vi "TimedTrigger.vi"(8 "error in (no error)":errorcluster, 10 "clTimedTrigger":T1={"TriggerName"="", "Time after next UTC Second"=0.0, "Trigger Duration"=0.1, "Edge"=enum."Rising"}, 11 "PXI_MultiTrig in":refnum<class "PXI_MultiTrig.lvclass">) -> (0 "error out":errorcluster, 3 "PXI_MultiTrig out":refnum<class "PXI_MultiTrig.lvclass">)   [LabVIEW 2018, in "SyncPlugins.lvlib" / "PXI_MultiTrig.lvclass"]
uses:
  PXI_MultiTrig.lvclass
  SyncPluginBase/Typedefs/clTimedTrigger.ctl
  PXI_MultiTrig.lvclass/PXI_MultiTrig.ctl
  Accessors/Read RefClkSession.vi
  Accessors/Write RefClkSession.vi
  Accessors/Write Triggers.vi
  Accessors/Read Triggers.vi
  <vilib>/Utility/error.llb/Error Cluster From Error Code.vi
  <vilib>/ErrorRing/Error Ring.xnode
  SyncPluginBase/SyncPluginBase.lvclass
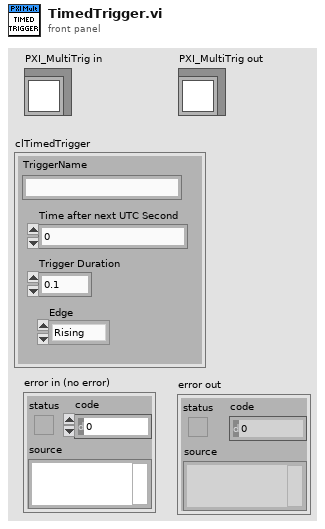
[diagram p1: front panel]
types:
  T1 = typedef "SyncPlugins.lvlib/SyncPluginBase.lvclass/clTimedTrigger.ctl" = cluster{"TriggerName":string, "Time after next UTC Second":dbl, "Trigger Duration":dbl, "Edge":enum16{"Rising", "Falling"}}
  T2 = typedef "SyncPlugins.lvlib/PXI_MultiTrig.lvclass/clTrigger.ctl" = cluster{"Name":string, "DestTerm":string, "SrcTerm":string, "SyncClk":string, "Edge":i32, "Invert?":i32, "Initiated":bool, "Type":string, "TrigTime":bool}
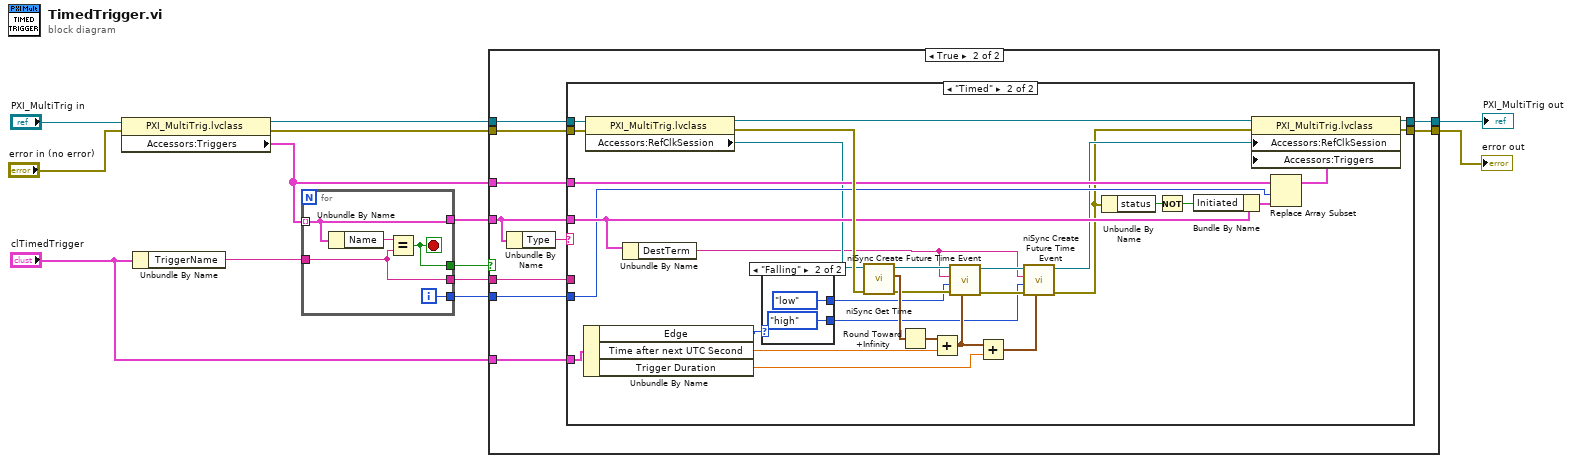
[diagram p0: block diagram]
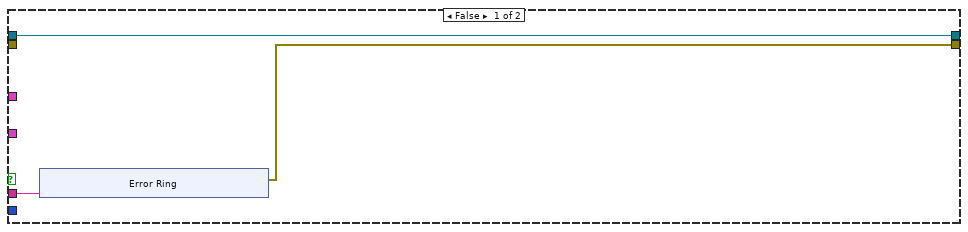
[diagram p2: hidden frame]
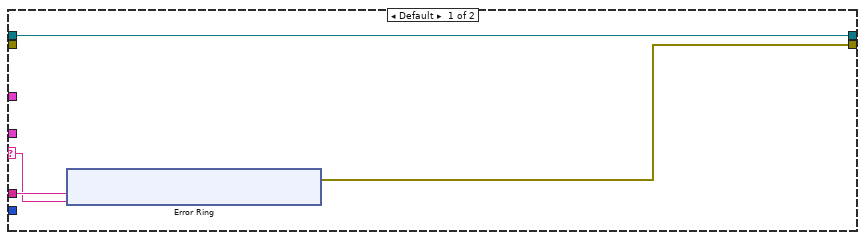
[diagram p3: hidden frame]
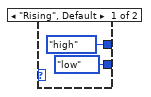
[diagram p4: hidden frame]
diagram:
  n1 = property class="PXI_MultiTrig.lvclass"(reference="PXI_MultiTrig in", error in="error in (no error)") -> (reference out=w8:refnum<class "PXI_MultiTrig.lvclass">, error out=w7:errorcluster, "Accessors:Triggers"=w2:T2[])
  n2 = Unbundle By Name("clTimedTrigger") -> ("TriggerName"=w11:string)
  n3 = for {
    tunnel: w2 -> [w17] mode=indexing
    tunnel: w11 -> [w15]
    tunnel: [w17] -> w4
    tunnel: [w16] -> w10
    tunnel: [w15] -> w9
    tunnel: [w14] -> w3
    i -> [w14]
    stop <- w16 stop-if-true
    n4 = Unbundle By Name(w17) -> ("Name"=w18:string)
    n5 = Equal?(x=w18, y=w15) -> (x = y?=w16:bool)
  }
  n6 = case shown="True" w10 {
    tunnel: w9 -> [w21 w37]
    tunnel: w8 -> [w20 w32]
    tunnel: w7 -> [_ w30]
    tunnel: [w20 w31] -> w6
    tunnel: [w19 w34] -> w5
    tunnel: w4 -> [_ w33]
    tunnel: w3 -> [_ w36]
    tunnel: w2 -> [_ w35]
    tunnel: "clTimedTrigger" -> [_ w29]
    frame False {
      n7 = xnode "Error Ring"("parameter 0"=w21) -> ("error out"=w19:errorcluster)
    }
    frame True {
      n8 = Unbundle By Name(w33) -> ("Type"=w38:string)
      n9 = case shown="\"Timed\"" w38 {
        selector: w38 -> [w41 _]
        tunnel: w37 -> [w42 _]
        tunnel: w36 -> [_ w67]
        tunnel: w35 -> [_ w68]
        tunnel: [w40 w73] -> w34
        tunnel: w33 -> [_ w72]
        tunnel: w32 -> [w39 w80]
        tunnel: [w39 w74] -> w31
        tunnel: w30 -> [_ w81]
        tunnel: w29 -> [_ w56]
        frame Default {
          n10 = xnode "Error Ring"("parameter 0"=w42, "parameter 1"=w41) -> ("error out"=w40:errorcluster)
        }
        frame "Timed" {
          n11 = Unbundle By Name(w56) -> ("Edge"=w53:enum16{"Rising", "Falling"}, "Time after next UTC Second"=w55:dbl, "Trigger Duration"=w54:dbl)
          n12 = property class="PXI_MultiTrig.lvclass"(reference=w80, error in=w81) -> (reference out=w75:refnum<class "PXI_MultiTrig.lvclass">, error out=w79:errorcluster, "Accessors:RefClkSession"=w65:refnum<k15>)
          n13 = Unbundle By Name(w72) -> ("DestTerm"=w59:string)
          n14 = case shown="\"Falling\"" w53 {
            tunnel: [enum32{"low", "high"}."low" ("output level") enum32{"low", "high"}."high" ("output level")] -> w52
            tunnel: [enum32{"low", "high"}."high" ("output level") enum32{"low", "high"}."low" ("output level")] -> w51
            frame "Rising", Default {
            }
            frame "Falling" {
            }
          }
          n15 = call <instrlib>:"niSync Get Time.vi"("error in (no error)"=w79, "instrument handle"=w65) -> ("error out"=w76:errorcluster, "time"=w78:timestamp, "instrument handle out"=w64:refnum<k15>)  [unwired: 5 in]
          n16 = Round Toward +Infinity(x=w78) -> (ceil(x): smallest int >= x=w77:timestamp)
          n17 = Add(x=w77, y=w55) -> (x+y=w61:timestamp)
          n18 = call <instrlib>:"niSync Create Future Time Event.vi"("time"=w61, "error in (no error)"=w76, "output level"=w51, "terminal"=w59, "instrument handle"=w64) -> ("error out"=w63:errorcluster, "instrument handle out"=w62:refnum<k15>)  [unwired: 4 in]
          n19 = Add(x=w61, y=w54) -> (x+y=w60:timestamp)
          n20 = call <instrlib>:"niSync Create Future Time Event.vi"("time"=w60, "error in (no error)"=w63, "output level"=w52, "terminal"=w59, "instrument handle"=w62) -> ("error out"=w57:errorcluster, "instrument handle out"=w58:refnum<k15>)  [unwired: 4 in]
          n21 = Unbundle By Name(w57) -> ("status"=w71:bool)
          n22 = Not(x=w71) -> (.not. x?=w70:bool)
          n23 = Bundle By Name(cluster=w72, "Initiated"=w70) -> (w69:T2)
          n24 = Replace Array Subset(array=w68, new element=w69, index=w67) -> (w66:T2[])
          n25 = property class="PXI_MultiTrig.lvclass"(reference=w75, error in=w57, "Accessors:RefClkSession"=w58, "Accessors:Triggers"=w66) -> (reference out=w74:refnum<class "PXI_MultiTrig.lvclass">, error out=w73:errorcluster)
        }
      }
    }
  }
  "error out" <- w5
  "PXI_MultiTrig out" <- w6
